vi "Get NumOfComponent.vi"(8 "error in (no error)":errorcluster, 11 "BrowerComposite in":refnum<class "BrowerComposite.lvclass">) -> (0 "error out":errorcluster, 2 "NumOfItems":i32, 3 "BrowerComposite out":refnum<class "BrowerComposite.lvclass">)   [LabVIEW 2015, in "BrowerComposite.lvclass"]
uses:
  BrowerComposite.lvclass
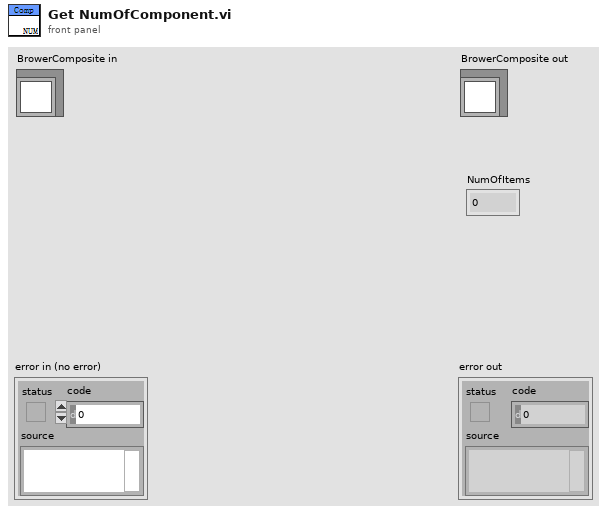
[diagram p1: front panel]
types:
  T1 = typedef "BrowerComposite.lvclass/ObjectAttributes.ctl" = cluster{"BrowerComponents":refnum<class "BrowerComponent.lvclass">[], "BrowerComponentIDs":string[], "Iterator":refnum<class "Iterator.lvclass">}
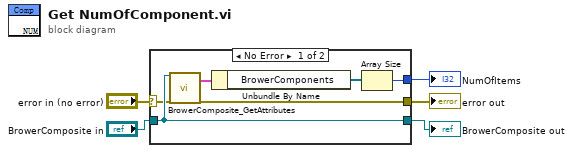
[diagram p0: block diagram]
diagram:
  n1 = case shown="No Error" "error in (no error)" {
    selector: "error in (no error)" -> [w10 w13]
    tunnel: [w9 w13] -> w4
    tunnel: [w11 w12] -> w2
    tunnel: "BrowerComposite in" -> [w11 w12]
    tunnel: [w6 _] -> w1
    frame No Error {
      n2 = call "BrowerComposite_GetAttributes.vi"("reference in"=w11, "error in (no error)"=w10) -> ("Data"=w8:T1, "error out"=w9:errorcluster)  [unwired: 14 in, 2 out]
      n3 = Unbundle By Name(w8) -> ("BrowerComponents"=w7:refnum<class "BrowerComponent.lvclass">[])
      n4 = Array Size(array=w7) -> (size(s)=w6:i32)
    }
    frame Error {
    }
  }
  "error out" <- w4
  "BrowerComposite out" <- w2
  "NumOfItems" <- w1
